vi "Boolean Latch.vi"(1 "Input":bool, 2 "Reset":bool) -> (0 "Output":bool)   [LabVIEW 2015]
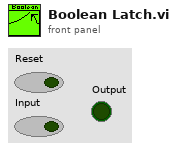
[diagram p1: front panel]
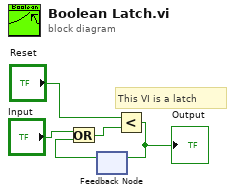
[diagram p0: block diagram]
diagram:
  # "This VI is a latch"
  n1 = feedback #1() -> (w2:bool)  [unwired: 1 in]
  n2 = Or(x="Input", y=w2) -> (x .or. y?=w1:bool)
  n3 = Less?(x="Reset", y=w1) -> (x < y?=w3:bool)
  "Output" <- w3
  n4 = feedback-in #1(w3) -> ()
